vi "SIM Generate Adams Coeffs.vi"(0 "Max Order":i32=15) -> (1 "AB Coefficients":dbl[](array[numeric])=[1.0, 0.5, 0.4166666666666667, 0.375, 0.34861111111111115, 0.32986111111111116, 0.3155919312169312, 0.3042245370370372, 0.29486800044091704, 0.2869754464285714, 0.2801895964439367, 0.2742655400315989, 0.2690288467736488, 0.26435134836660656, 0.26013639612760103], 2 "AM Coefficients":dbl[](array[numeric])=[1.0, -0.5, -0.08333333333333331, -0.041666666666666685, -0.026388888888888906, -0.01874999999999996, -0.014269179894179918, -0.011367394179894186, -0.009356536596119916, -0.00789255401234569, -0.006785849984634704, -0.005924056412337661, -0.005236693257950287, -0.004677498407042249, -0.004214952239005483])   [LabVIEW 2020]
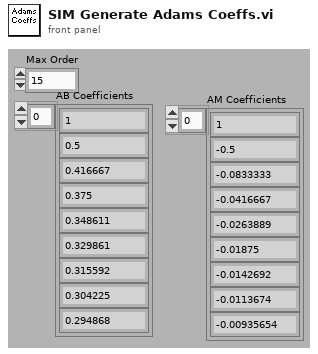
[diagram p1: front panel]
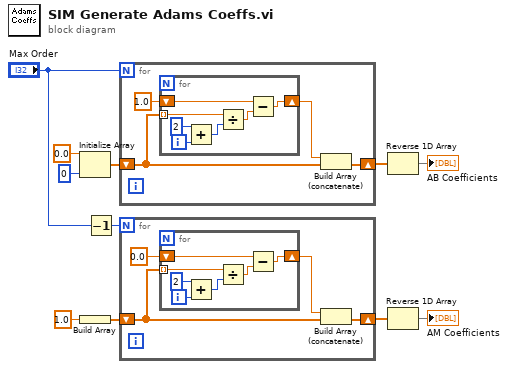
[diagram p0: block diagram]
diagram:
  n1 = Initialize Array(0.0 ("element"), 0 ("dimension size")) -> (w11:dbl[])
  n2 = Build Array(1.0) -> (w3:dbl[])
  n3 = Decrement(x="Max Order") -> (x-1=w2:i32)
  n4 = for {
    N: "Max Order" -> [_]
    shift-right: [w15] -> w8
    shift-left: w11 -> [w14]
    n5 = for {
      shift-right: [w19] -> w12
      shift-left: 1.0 -> [w17]
      tunnel: w14 -> [w16] mode=indexing
      i -> [w21]
      n6 = Add(x=2, y=w21) -> (x+y=w20:i32)
      n7 = Divide(x=w16, y=w20) -> (x/y=w18:dbl)
      n8 = Subtract(x=w17, y=w18) -> (x-y=w19:dbl)
    }
    n9 = Build Array (concatenate)(w12, w14) -> (w15:dbl[])
  }
  n10 = for {
    N: w2 -> [_]
    shift-right: [w26] -> w6
    shift-left: w3 -> [w25]
    n11 = for {
      shift-right: [w30] -> w24
      shift-left: 0.0 ("element") -> [w28]
      tunnel: w25 -> [w27] mode=indexing
      i -> [w32]
      n12 = Add(x=2, y=w32) -> (x+y=w31:i32)
      n13 = Divide(x=w27, y=w31) -> (x/y=w29:dbl)
      n14 = Subtract(x=w28, y=w29) -> (x-y=w30:dbl)
    }
    n15 = Build Array (concatenate)(w24, w25) -> (w26:dbl[])
  }
  n16 = Reverse 1D Array(array=w8) -> (reversed array=→"AB Coefficients":dbl[])
  n17 = Reverse 1D Array(array=w6) -> (reversed array=→"AM Coefficients":dbl[])
